vi "未命名 1.vi"() -> ()   [LabVIEW 2013]
panel:
  in  "数组":u16[][](array[numeric])
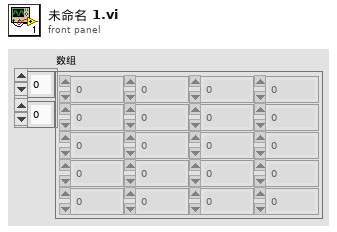
[diagram p1: front panel]
types:
  T1 = typedef "IMAQ Image.ctl" = refnum<image>
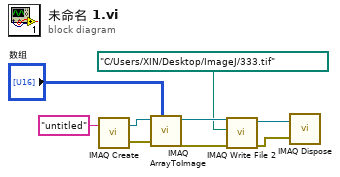
[diagram p0: block diagram]
diagram:
  n1 = call "IMAQ Create"("Image Name"="untitled") -> ("New Image"=w3:T1, "error out"=w2:errorcluster)  [unwired: 4 in]
  n2 = call "IMAQ ArrayToImage"("Image Pixels (U16)"="数组", "error in (no error)"=w2, "Image"=w3) -> ("error out"=w5:errorcluster, "Image Out"=w8:T1)  [unwired: 7 in]
  n3 = call-poly "IMAQ Write File 2"("error in (no error)"=w5, "File Path"=path "C:/Users/XIN/Desktop/ImageJ/333.tif", "Image"=w8) -> ("error out"=w6:errorcluster, "Image Out (duplicate)"=w7:T1)  [unwired: 7 in]
  n4 = call "IMAQ Dispose"("Image"=w7, "error in (no error)"=w6) -> ()  [unwired: 4 in, 1 out]
